vi "Save Prefs.vi"(8 "error in (no error)":errorcluster, 11 "PrefsDB in":refnum<class "PrefsDB.lvclass">) -> (0 "error out":errorcluster, 3 "PrefsDB out":refnum<class "PrefsDB.lvclass">)   [LabVIEW 2020, in "User Prefs.lvlib" / "PrefsDB.lvclass"]
uses:
  PrefsDB.lvclass
  PrefsDB.lvclass/PrefsDB.ctl
  lv-cdm/CDM-Config/Config-JSON/Config-JSON.lvclass
  C:/dev/lv20CE/relink/lv-cdm/CDM-Config/Config Storage/Config Storage.lvclass
  lv-cdm/CDM-Config/Config Storage/Config Storage.lvclass
  lv-cdm/CDM-Config/Config Manager/Config Manager.lvclass
  lv-cdm/CDM-Config/Config Element/Config Element.lvclass
  C:/dev/lv20CE/relink/lv-cdm/CDM-Config/Config-JSON/Config-JSON.lvclass
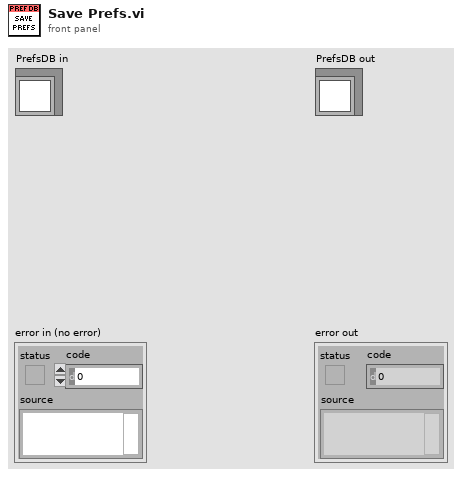
[diagram p1: front panel]
types:
  T1 = typedef "User Prefs.lvlib/PrefsDB.lvclass/Ref Data.ctl" = cluster{"Map":map{string, T2}}
  T2 = typedef "User Prefs.lvlib/PrefsDB.lvclass/Pref Group.ctl" = cluster{"Config Manager":refnum<class "Config Manager.lvclass">, "Group":string}
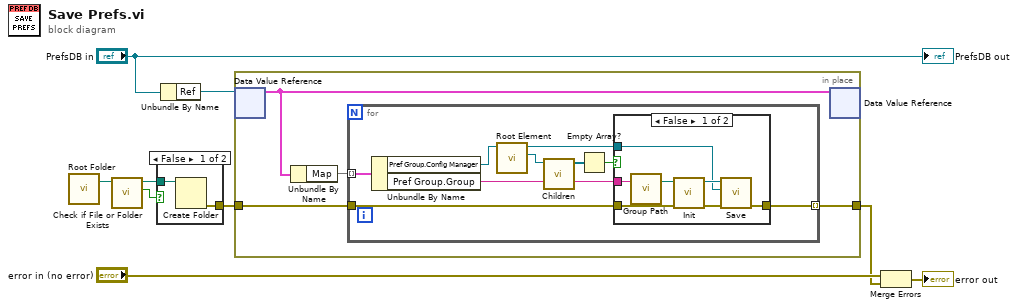
[diagram p0: block diagram]
diagram:
  n1 = call "Root Folder.vi"() -> ("Prefs Root"=w4:path)  [unwired: 7 in]
  n2 = call <vilib>:"Check if File or Folder Exists.vi"("path"=w4) -> ("file or folder exists?"=w3:bool, "dup path"=w2:path)  [unwired: 8 in, 1 out]
  n3 = case shown="False" w3 {
    tunnel: w2 -> [w11 _]
    tunnel: [w10 _] -> w1
    frame False {
      n4 = Create Folder(path (use dialog)=w11) -> (error out=w10:errorcluster)  [unwired: 2 in, 2 out]
    }
    frame True {
    }
  }
  n5 = Unbundle By Name("PrefsDB in") -> ("Ref"=w7:refnum<data-value>)
  n6 = in-place {
    in-place-border: [w14] -> w5
    in-place-border: w1 -> [w12]
    n7 = in-place-dvr #1(w7) -> (w13:T1)  [unwired: 1 out]
    n8 = Unbundle By Name(w13) -> ("Map"=w15:map{string, T2})
    n9 = for {
      tunnel: w15 -> [w24] mode=indexing
      tunnel: [w23] -> w14 mode=indexing
      tunnel: w12 -> [w21]
      n10 = Unbundle By Name(w24) -> ("Pref Group.Config Manager"=w20:refnum<class "Config Manager.lvclass">, "Pref Group.Group"=w22:string)
      n11 = call "Root Element.vi"("Config Manager in"=w20) -> ("Root Element"=w19:refnum<class "Config Element.lvclass">, "Config Manager out"=w16:refnum<class "Config Manager.lvclass">)  [unwired: 8 in, 1 out]
      n12 = call "Children.vi"("Config Element in"=w19) -> ("Elements"=w18:refnum<class "Config Element.lvclass">[])  [unwired: 9 in, 1 out]
      n13 = Empty Array?(array=w18) -> (empty?=w17:bool)
      n14 = case shown="False" w17 {
        tunnel: [w29 w32] -> w23
        tunnel: w22 -> [w28 _]
        tunnel: w21 -> [w26 w32]
        tunnel: w16 -> [w25 _]
        frame False {
          n15 = call "Group Path.vi"("Group Name"=w28) -> ("Group Path"=w27:path)  [unwired: 6 in]
          n16 = call "Init.vi"("error in (no error)"=w26, "Path"=w27) -> ("error out"=w30:errorcluster, "Config-JSON out"=w31:refnum<class "Config-JSON.lvclass">)  [unwired: 8 in]
          n17 = call "Save.vi"("error in (no error)"=w30, "Config"=w25, "Config Storage in"=w31) -> ("error out"=w29:errorcluster)  [unwired: 7 in, 1 out]
        }
        frame True {
          # "Nothing to save"
        }
      }
    }
    n18 = in-place-dvr #1(w13) -> ()  [unwired: 2 out]
  }
  n19 = Merge Errors("error in (no error)", w5) -> (→"error out":errorcluster)
  "PrefsDB out" <- "PrefsDB in"
